vi "TestWebVI.vi"() -> ()   [LabVIEW 2017]
uses:
  <vilib>/addons/InsightCM/Devices/Shared/WebDeviceResources/InternalInterface/controls/DataStoreAction.ctl
  <vilib>/addons/InsightCM/Devices/Shared/TransceiverComm/controls/TransComm_ConnectionInfo.ctl
  <vilib>/addons/InsightCM/Devices/Shared/cRIOAutoDetectHW/RT/controls/cRIO Product Info.ctl
  <vilib>/addons/InsightCM/Devices/Shared/cRIOAutoDetectHW/RT/controls/SystemHW.ctl
  <vilib>/addons/InsightCM/Devices/Shared/RT Utility/ImageInfo/controls/FirmwareProperties.ctl
panel:
  in  "firmware properties":T1={"title"="testFW", "description"="123", "ID"="{GUID}", "version"="5.6.7.8"}
  in  "SystemHW":T2={"controller"={"vendorName"="NI", "productName"="NI 9068", "serialNumber"="asdffgdf"}, "chassis"={"vendorName"="NI", "productName"="NI 9068", "serialNumber"="asdfdgf"}, "modules"=[{"vendorName"="NI", "productName"="NI 9205", "serialNumber"="asdffggf"}, {"vendorName"="NI", "productName"="NI 9232", "serialNumber"="12345345"}]}
  in  "ConnectionInfo":T4={"ClientName"="jackTest", "TransceiverHost"="transceiver", "TransceiverPort"=6342, "Password"="helloworld"}
  in  "Stop Button":bool
  out "IterationCount":i32
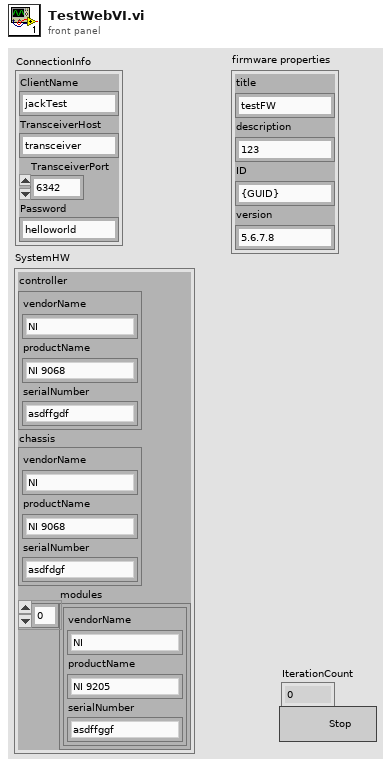
[diagram p1: front panel]
types:
  T1 = typedef "FirmwareProperties.ctl" = cluster{"title":string, "description":string, "ID":string, "version":string}
  T2 = typedef "SystemHW.ctl" = cluster{"controller":T3, "chassis":T3, "modules":T3[]}
  T3 = typedef "cRIO Product Info.ctl" = cluster{"vendorName":string, "productName":string, "serialNumber":string}
  T4 = typedef "TransComm_ConnectionInfo.ctl" = cluster{"ClientName":string, "TransceiverHost":string, "TransceiverPort":u16, "Password":string}
  T5 = typedef "WebDeviceResources.lvlib/DataStoreAction.ctl" = enum16{"Initialize", "Get", "Set"}
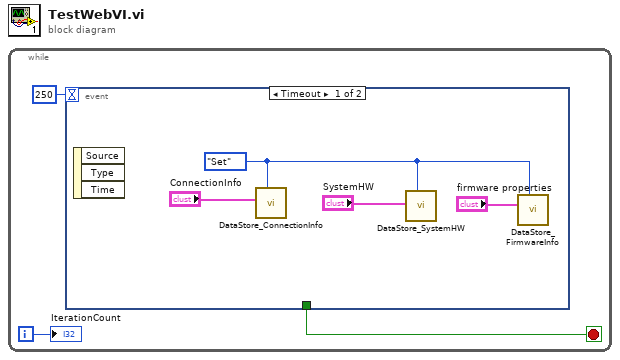
[diagram p0: block diagram]
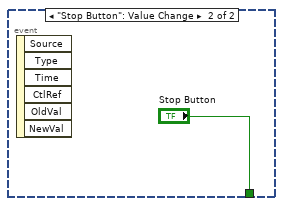
[diagram p2: hidden frame]
diagram:
  n1 = while {
    i -> [w1]
    stop <- w2 stop-if-true
    n2 = event shown="[0] Timeout" {
      selector: _ -> [_ _]
      dyn-events: _ -> [_ _]
      timeout: 250 -> [_ _]
      tunnel: [_ "Stop Button"] -> w2
      event Timeout {
        w5 = DataStoreAction."Set" ("Action")
        n3 = event-data() -> ()  [unwired: 1 in, 3 out]
        n4 = call <vilib>:"DataStore_ConnectionInfo.vi"("Action"=w5, "ConnInfo"="ConnectionInfo") -> ()  [unwired: 9 in, 1 out]
        n5 = call <vilib>:"DataStore_SystemHW.vi"("Action"=w5, "SystemHW"="SystemHW") -> ()  [unwired: 9 in, 1 out]
        n6 = call <vilib>:"DataStore_FirmwareInfo.vi"("Action"=w5, "Firmware Properties"="firmware properties") -> ()  [unwired: 9 in, 1 out]
      }
      event "Stop Button": Value Change {
        n7 = event-data() -> ()  [unwired: 1 in, 6 out]
      }
    }
    "IterationCount" <- w1
  }
